vi "finalize binding.vi"(8 "error in (no error)":errorcluster, 11 "SQLite3LV Cursor in":refnum<class "cursor.lvclass">) -> (0 "error out":errorcluster, 3 "SQLite3LV Cursor out":refnum<class "cursor.lvclass">)   [LabVIEW 2014, in "SQLite3LV.lvlib" / "cursor.lvclass"]
uses:
  cursor.lvclass
  cursor.lvclass/cursor.ctl
  sqlite3_64.dll
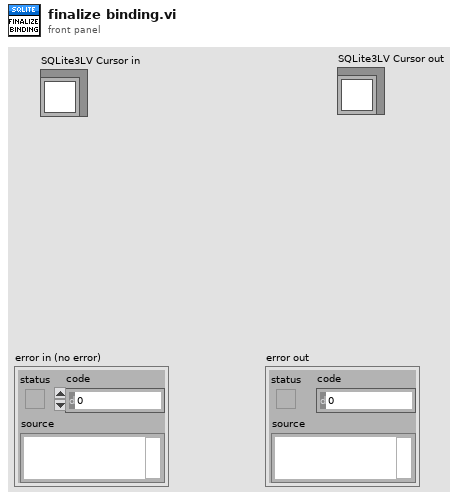
[diagram p1: front panel]
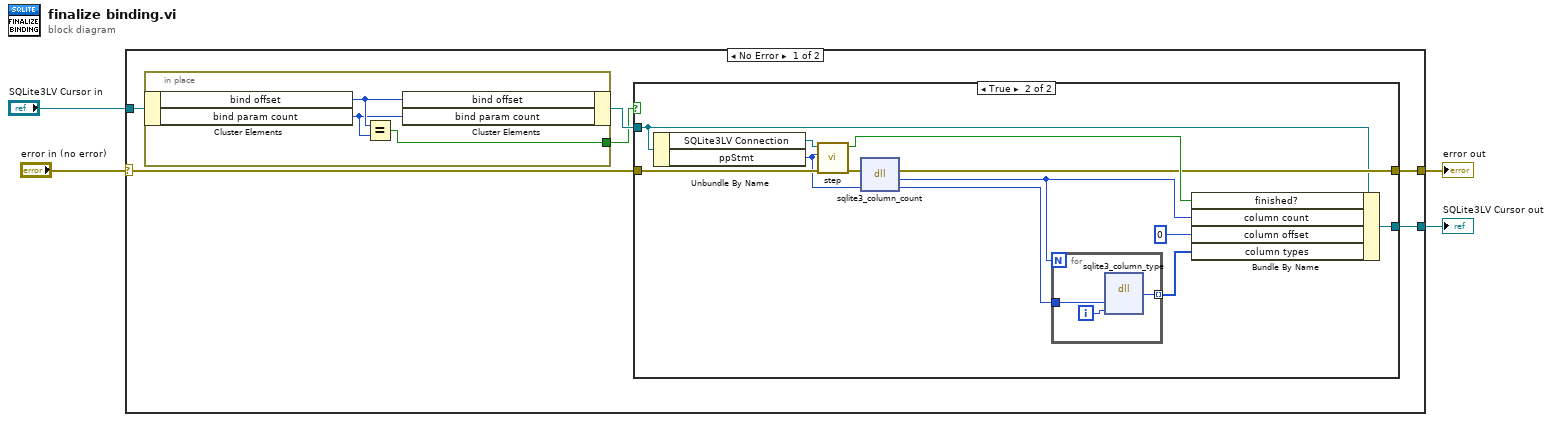
[diagram p0: block diagram]
diagram:
  n1 = case shown="No Error" "error in (no error)" {
    selector: "error in (no error)" -> [w9 w32]
    tunnel: [w10 w32] -> w4
    tunnel: "SQLite3LV Cursor in" -> [w7 w31]
    tunnel: [w8 w31] -> w1
    frame No Error {
      n2 = in-place {
        in-place-border: [w11] -> w5
        n3 = in-place-cluster #1(w7) -> ("bind offset"=w13:i32, "bind param count"=w12:i32)
        n4 = Equal?(x=w13, y=w12) -> (x = y?=w11:bool)
        n5 = in-place-cluster #1("bind offset"=w13, "bind param count"=w12) -> (w6:refnum<class "cursor.lvclass">)
      }
      n6 = case shown="True" w5 {
        tunnel: [w15 w22] -> w10
        tunnel: w9 -> [w15 w27]
        tunnel: w6 -> [w14 w18]
        tunnel: [w14 w26] -> w8
        frame False {
        }
        frame True {
          n7 = Unbundle By Name(w18) -> ("SQLite3LV Connection"=w17:refnum<class "sqlite3.lvclass">, "ppStmt"=w16:i64)
          n8 = call "step.vi"("error in (no error)"=w27, "pStmt"=w16, "psqlite"=w17) -> ("error out"=w24:errorcluster, "finished?"=w25:bool)  [unwired: 7 in]
          n9 = dll-call lib="C:/Users/BobUser/Desktop/LVTables/sqlite3**.*" fn="sqlite3_column_count"(error in=w24, "pStmt"=w16) -> (error out=w22:errorcluster, "column count"=w21:i32, "pStmt"=w20:i64)  [unwired: 2 in, 1 out]
          n10 = for {
            N: w21 -> [_]
            tunnel: w20 -> [w29]
            tunnel: [w28] -> w19 mode=indexing
            i -> [w30]
            n11 = dll-call lib="C:/Users/BobUser/Desktop/LVTables/sqlite3**.*" fn="sqlite3_column_type"("pStmt"=w29, "iCol"=w30) -> ("column type"=w28:i32)  [unwired: 5 in, 2 out]
          }
          n12 = Bundle By Name(cluster=w18, "finished?"=w25, "column count"=w21, "column offset"=0 ("active statement.column offset"), "column types"=w19) -> (w26:refnum<class "cursor.lvclass">)
        }
      }
    }
    frame Error {
    }
  }
  "error out" <- w4
  "SQLite3LV Cursor out" <- w1
